vi "REQ full lifecycle.vi"(0 "ZMQ endpoint":string="tcp://127.0.0.1:5555", 1 "Julia user functions script":path=path "dummy.jl", 2 "LV Client state in":T2, 5 "data to send":string="hello", 7 "ZMQ new Timeouts in":T1={"SNDTIMEO"=-1, "RCVTIMEO"=-1}, 9 "Force command":bool, 11 "error in":errorcluster, 12 "command":T3, 13 "Jl Server state in":T2) -> (3 "LV Client state out":T2, 4 "server response":string, 6 "socket out":refnum<class "zmq_socket.lvclass">, 8 "ZMQ timeouts out":cluster{"previous":T1, "current":T1}={"previous"={"SNDTIMEO"=-1, "RCVTIMEO"=-1}, "current"={"SNDTIMEO"=-1, "RCVTIMEO"=-1}}, 10 "timeout?":bool, 14 "Jl Server state out":T2, 15 "error out":errorcluster)   [LabVIEW 2018, in "LV2Julia_core.lvlib"]
doc: "This is the central piece of the package. The VI is based on Functional Global Variable pattern to keep book on the state of the Julia server and LabView client. See the available states of the \"command\" input. For some commands, the \"Force command\" must be set."
uses:
  LV2Julia_core.lvlib
  Commands.ctl
  Server or client state.ctl
  ZMQ timeouts.ctl
  <vilib>/addons/zeromq/zmq_socket.lvclass
  <vilib>/addons/zeromq/zmq_context.lvclass
  commands LV2Jl.ctl
  expected server response.ctl
  <vilib>/addons/zeromq/socket_options.ctl
  <vilib>/Utility/error.llb/Error Cluster From Error Code.vi
  ZMQ timeouts global.vi
  <vilib>/addons/zeromq/zmq_getsocketopt_int.vi
  <vilib>/ErrorRing/Error Ring.xnode
  <vilib>/addons/zeromq/zeromq.lvlib
panel:
  out "return code":i32
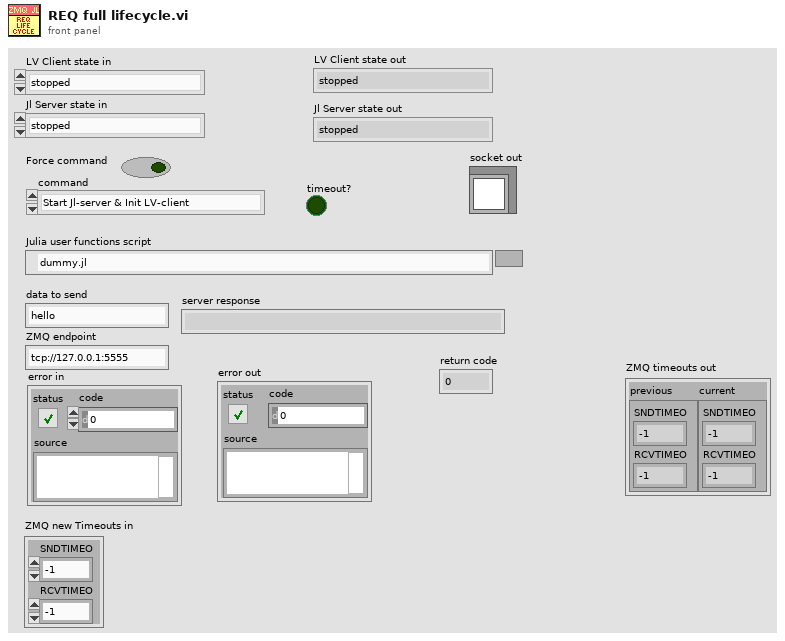
[diagram p1: front panel]
types:
  T1 = typedef "LV2Julia_core.lvlib/ZMQ timeouts.ctl" = cluster{"SNDTIMEO":i32, "RCVTIMEO":i32}
  T2 = typedef "LV2Julia_core.lvlib/Server or client state.ctl" = enum16{"stopped", "running", "unknown"}
  T3 = typedef "LV2Julia_core.lvlib/Commands.ctl" = enum16{"Start Jl-server & Init LV-client", "Send request & Get response ", "Stop Jl-server & Cleanup LV-client", "Cleanup LV-client", "Start Jl-server", "Stop Jl-server", "Init LV-Client", "Cleanup LV-Client", "(not allowed)", "Set LV Client state", "Set Jl Server state", "set ZMQ timeout", "read ZMQ timeout", "read-out state"}
  T4 = typedef "zeromq.lvlib/socket_options.ctl" = enum8{"NONE", "ZMQ_HWM", "<2>", "ZMQ_SWAP", "ZMQ_AFFINITY", "ZMQ_IDENTITY", "ZMQ_SUBSCRIBE", "ZMQ_UNSUBSCRIBE", "ZMQ_RATE", "ZMQ_RECOVERY_IVL", "ZMQ_MCAST_LOOP", "ZMQ_SNDBUF", "ZMQ_RCVBUF", "ZMQ_RCVMORE", "ZMQ_FD", "ZMQ_EVENTS", "ZMQ_TYPE", "ZMQ_LINGER", "ZMQ_RECONNECT_IVL", "ZMQ_BACKLOG", "ZMQ_RECOVERY_IVL_MSEC", "ZMQ_RECONNECT_IVL_MAX", "ZMQ_MAXMSGSIZE", "ZMQ_SNDHWM", "ZMQ_RCVHWM", "ZMQ_MULTICAST_HOPS", "<26>", "ZMQ_RCVTIMEO", "ZMQ_SNDTIMEO", "<29>", "<30>", "ZMQ_IPV4ONLY", "ZMQ_LAST_ENDPOINT", "ZMQ_ROUTER_MANDATORY", "ZMQ_TCP_KEEPALIVE", "ZMQ_TCP_KEEPALIVE_CNT", "ZMQ_TCP_KEEPALIVE_IDLE", "ZMQ_TCP_KEEPALIVE_INTVL", "ZMQ_TCP_ACCEPT_FILTER", "ZMQ_DELAY_ATTACH_ON_CONNECT", "ZMQ_XPUB_VERBOSE"}
  T5 = typedef "LV2Julia_core.lvlib/expected server response.ctl" = u16
  T6 = typedef "LV2Julia_core.lvlib/commands LV2Jl.ctl" = u8
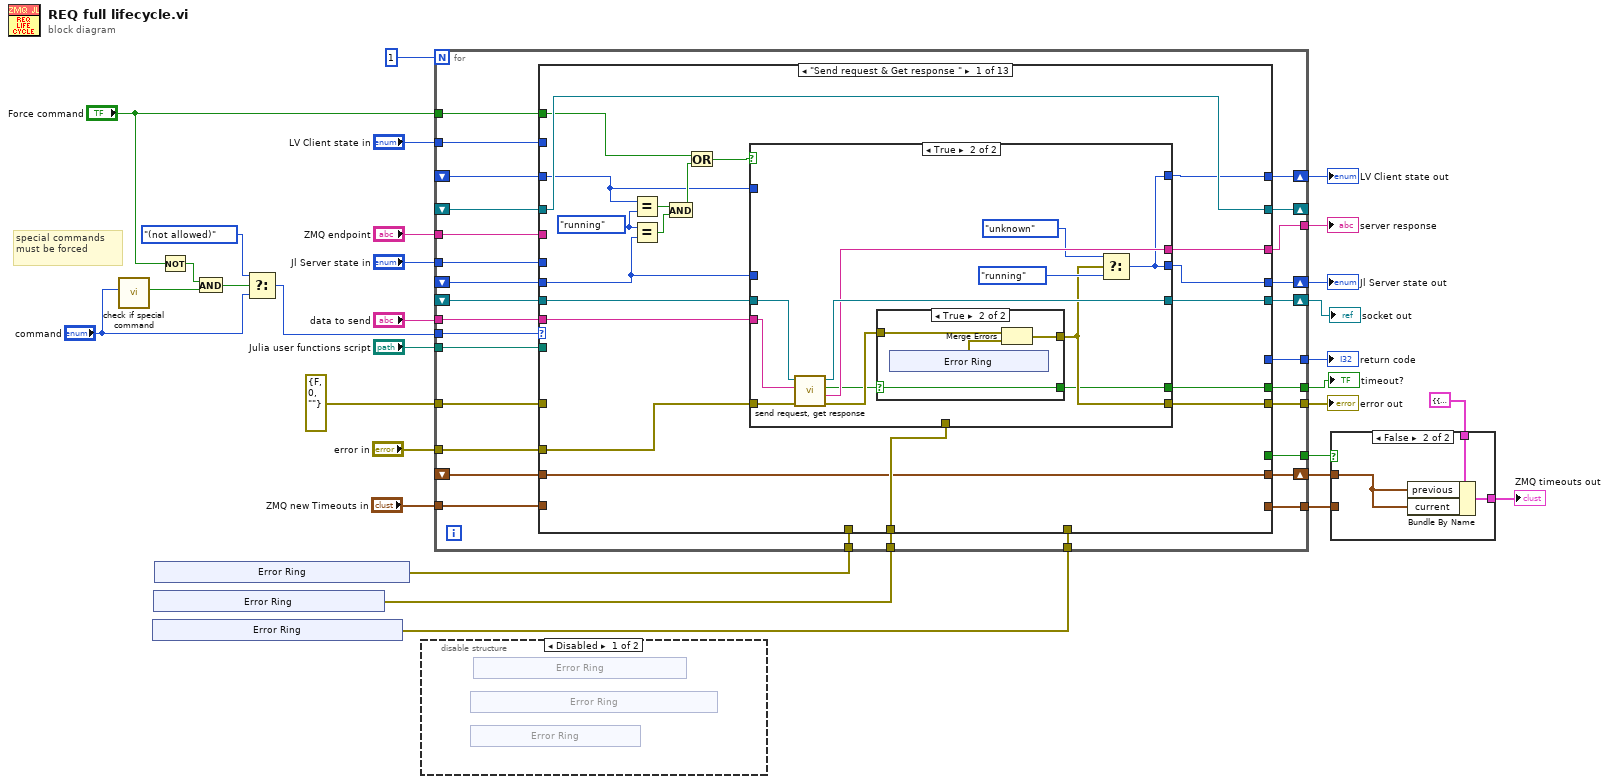
[diagram p0: block diagram]
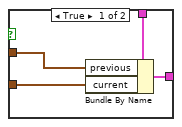
[diagram p2: hidden frame]
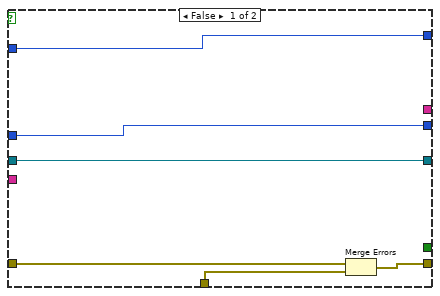
[diagram p4: hidden frame]
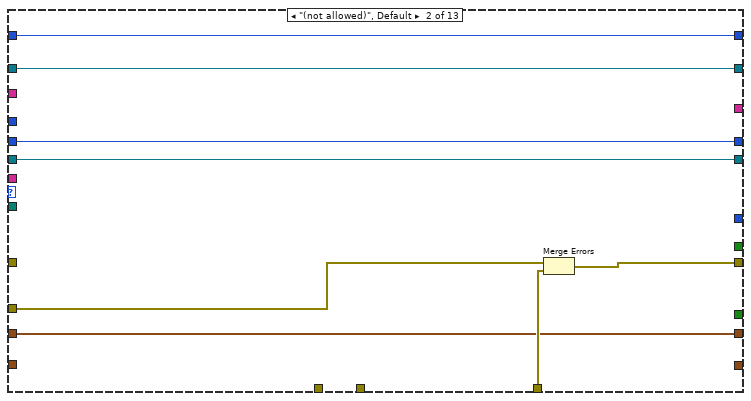
[diagram p6: hidden frame]
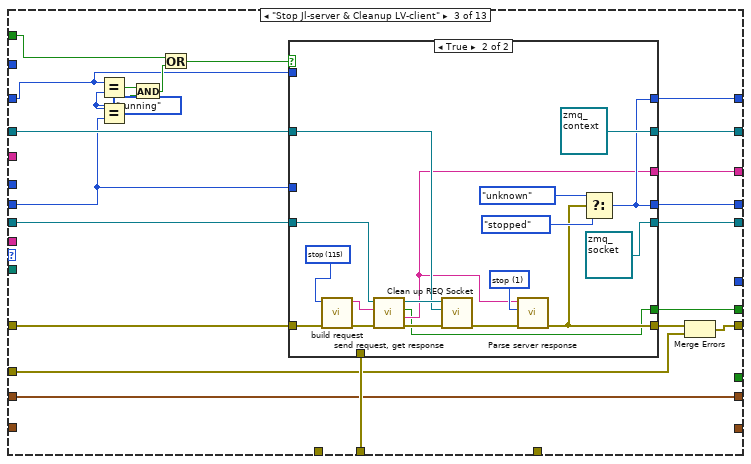
[diagram p7: hidden frame]
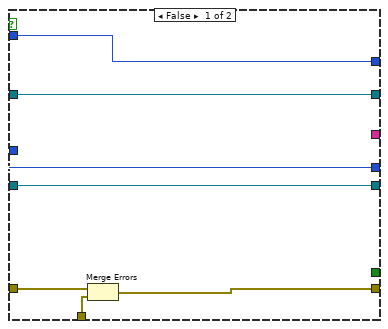
[diagram p8: hidden frame]
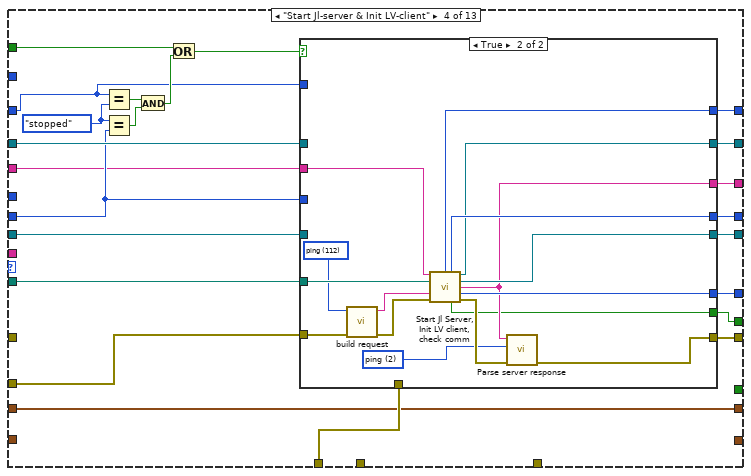
[diagram p9: hidden frame]
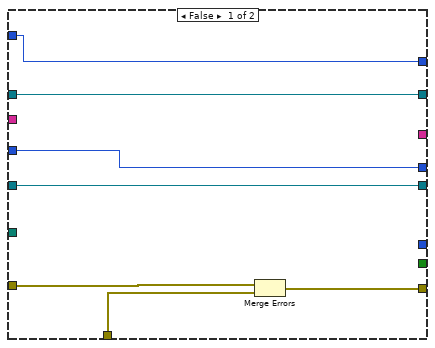
[diagram p10: hidden frame]
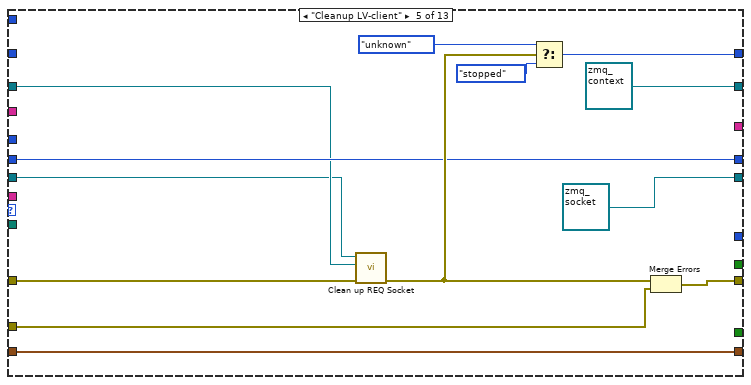
[diagram p11: hidden frame]
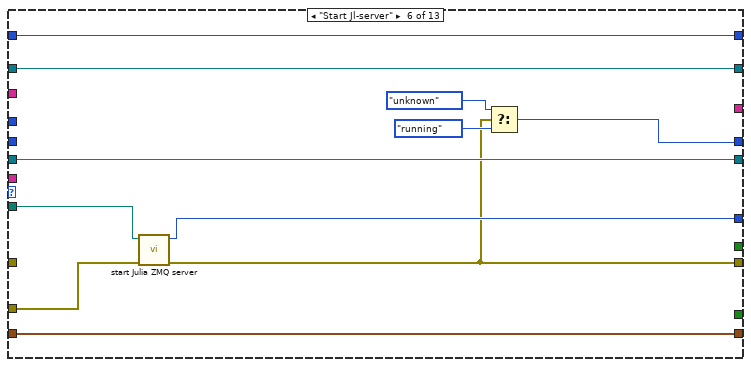
[diagram p12: hidden frame]
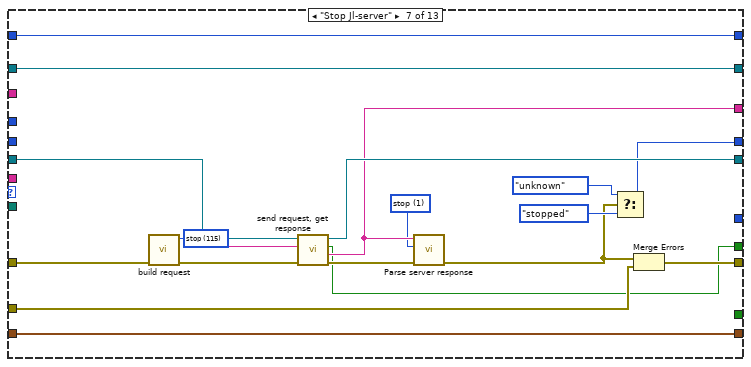
[diagram p13: hidden frame]
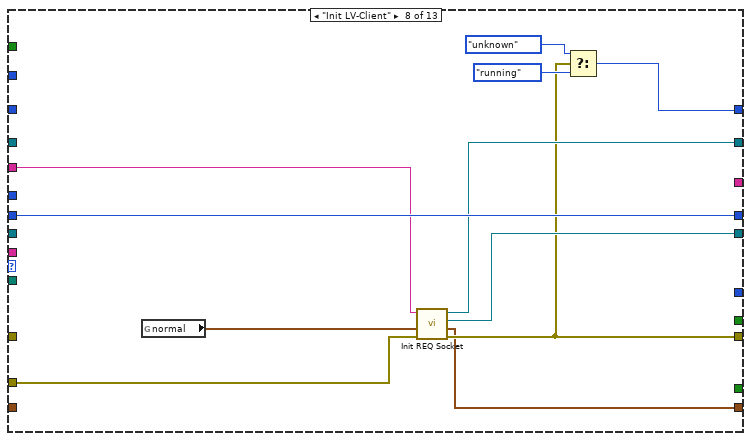
[diagram p14: hidden frame]
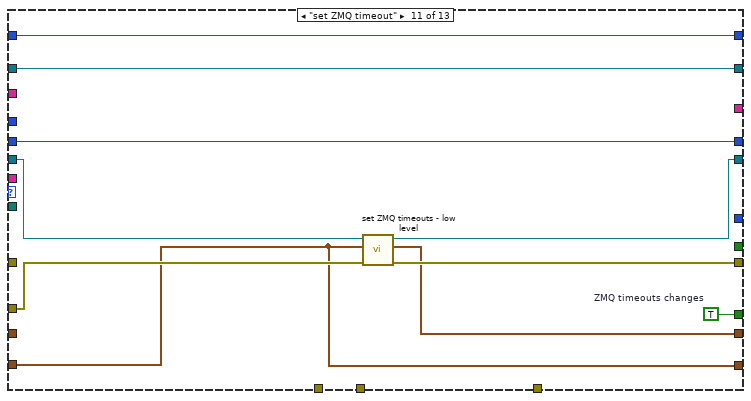
[diagram p17: hidden frame]
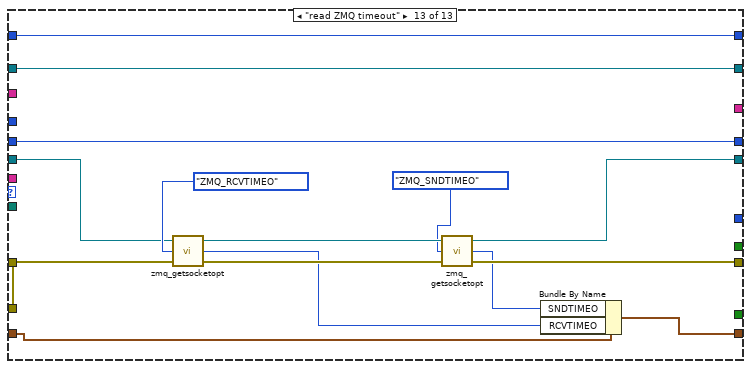
[diagram p19: hidden frame]
diagram:
  # "special commands must be forced"
  n1 = call "check if special command.vi"("command"="command") -> ("is special CMD"=w6:bool)  [unwired: 10 in]
  n2 = xnode "Error Ring"() -> ("error out"=w16:errorcluster)
  n3 = xnode "Error Ring"() -> ("error out"=w22:errorcluster)
  n4 = xnode "Error Ring"() -> ("error out"=w24:errorcluster)
  n5 = Not(x="Force command") -> (.not. x?=w20:bool)
  n6 = And(x=w20, y=w6) -> (x .and. y?=w19:bool)
  n7 = Select(t=Commands."(not allowed)" ("command"), s=w19, f="command") -> (s? t:f=w17:T3)
  n8 = disable-structure shown="Disabled" {
    frame Disabled {
      n9 = xnode "Error Ring"() -> ()  [unwired: 1 out]
      n10 = xnode "Error Ring"() -> ()  [unwired: 1 out]
      n11 = xnode "Error Ring"() -> ()  [unwired: 1 out]
    }
    frame Enabled {
    }
  }
  n12 = for {
    N: 1 -> [_]
    tunnel: [w75] -> w30
    tunnel: [w74] -> w29
    shift-right: [w73] -> _
    shift-left: _ -> [w66]
    tunnel: "ZMQ endpoint" -> [w72]
    tunnel: "data to send" -> [w71]
    shift-right: [w70] -> w9
    shift-left: _ -> [w65]
    tunnel: "error in" -> [w69]
    shift-right: [w67] -> w23
    shift-left: _ -> [w68]
    tunnel: w17 -> [w64]
    tunnel: "Julia user functions script" -> [w63]
    tunnel: w24 -> [w62]
    tunnel: "Force command" -> [w61]
    shift-right: [w60] -> w15
    shift-left: _ -> [w59]
    tunnel: w22 -> [w58]
    tunnel: w16 -> [w57]
    tunnel: [w56] -> w14
    tunnel: "LV Client state in" -> [w55]
    tunnel: "Jl Server state in" -> [w54]
    tunnel: errorcluster {"status"=FALSE, "code"=0, "source"=""} ("error in") -> [w53]
    tunnel: "ZMQ new Timeouts in" -> [w52]
    tunnel: [w50] -> w8
    shift-right: [w51] -> w4
    shift-left: _ -> [w49]
    tunnel: [w48] -> w3
    tunnel: [w47] -> w2
    n13 = case shown="\"Send request & Get response \"" w64 {
      tunnel: [w89 w131 w137 w201 w229 w241 w258 w272 w282 w288 w298 w302 w316] -> w75
      tunnel: [w90 _ w153 w190 _ _ w253 _ _ _ _ _ _] -> w74
      tunnel: [w95 w128 w148 w198 refnum<class "zmq_context.lvclass"> refnum ("zmq_context out") w246 w266 w274 w285 w290 w300 w306 w321] -> w73
      tunnel: w72 -> [_ _ _ w189 _ _ _ w271 _ _ _ _ _]
      tunnel: w71 -> [w91 _ _ _ _ _ _ _ _ _ _ _ _]
      tunnel: [w93 w126 w149 w194 refnum<class "zmq_socket.lvclass"> refnum ("zmq_socket out") w245 w265 w273 w283 w289 w295 w304 w317] -> w70
      tunnel: w69 -> [w94 w132 w136 w202 w227 w248 w256 w275 w282 w288 w297 w302 w314]
      tunnel: [w88 w127 w152 w197 w234 w242 w262 w277 w284 w287 w299 w305 w320] -> w67
      tunnel: w63 -> [_ _ _ w196 _ w239 _ _ _ _ _ _ _]
      tunnel: w65 -> [w92 w126 w154 w195 w232 w245 w268 _ w283 w289 w294 w304 w309]
      tunnel: w66 -> [w95 w128 w150 w199 w233 w246 w266 _ w285 w290 w300 w306 w321]
      tunnel: w68 -> [w79 w127 w141 w193 w234 _ _ w277 w284 _ w299 w305 w320]
      tunnel: w62 -> [_ _ _ w200 _ _ _ _ _ _ _ _ _]
      tunnel: w61 -> [w82 _ w142 w191 _ _ _ _ _ _ _ _ _]
      tunnel: [w87 w129 w140 w188 w235 w249 w267 w276 w281 w291 w301 w307 w322] -> w60
      tunnel: w59 -> [w80 w129 w138 w183 _ w249 w267 _ _ w291 w301 w307 w322]
      tunnel: w58 -> [w78 _ w139 _ _ _ _ _ _ _ _ _ _]
      tunnel: w57 -> [_ w130 _ _ _ _ _ _ _ _ _ _ _]
      tunnel: [_ _ _ w182 _ w247 _ _ _ _ _ _ _] -> w56
      tunnel: w55 -> [_ _ _ _ _ _ _ _ w281 _ _ _ _]
      tunnel: w54 -> [_ _ _ _ _ _ _ _ _ w287 _ _ _]
      tunnel: w53 -> [_ _ w135 _ w228 _ w257 _ _ _ _ _ _]
      tunnel: w52 -> [_ _ _ _ _ _ _ _ _ _ w292 _ _]
      tunnel: [w76 w125 w133 w180 w226 w240 w250 w270 w280 w286 w296 w303 w312] -> w51
      tunnel: [w77 _ w134 w181 _ _ w251 _ _ _ _ _ _] -> w50
      tunnel: w49 -> [w76 w125 w133 w180 w226 w240 w250 _ w280 w286 _ w303 w308]
      tunnel: [_ _ _ _ _ _ _ _ _ _ w293 _ _] -> w47
      tunnel: [_ _ _ _ _ _ _ _ _ _ w292 _ _] -> w48
      frame "Send request & Get response " {
        w85 = Server_or_client_state."running" ("Server state")
        n14 = Equal?(x=w80, y=w85) -> (x = y?=w83:bool)
        n15 = Equal?(x=w85, y=w79) -> (x = y?=w86:bool)
        n16 = And(x=w83, y=w86) -> (x .and. y?=w84:bool)
        n17 = Or(x=w82, y=w84) -> (x .or. y?=w81:bool)
        n18 = case shown="True" w81 {
          tunnel: w94 -> [w98 w113]
          tunnel: [w99 w112] -> w93
          tunnel: w92 -> [w99 w111]
          tunnel: w91 -> [_ w110]
          tunnel: [_ w109] -> w90
          tunnel: [w97 w104] -> w89
          tunnel: [w100 w106] -> w88
          tunnel: w79 -> [w100 _]
          tunnel: [w101 w106] -> w87
          tunnel: w80 -> [w101 _]
          tunnel: w78 -> [w96 _]
          tunnel: [_ w102] -> w77
          frame False {
            n19 = Merge Errors(w98, w96) -> (w97:errorcluster)
          }
          frame True {
            n20 = call "send request, get response.vi"("error in (no error)"=w113, "request"=w110, "zmq_socket in"=w111) -> ("error out"=w107:errorcluster, "response"=w109:string, "timeout?"=w103:bool, "zmq_socket out"=w112:refnum<class "zmq_socket.lvclass">)  [unwired: 4 in, 1 out]
            n21 = case shown="True" w103 {
              selector: w103 -> [w114 w116]
              tunnel: w107 -> [w115 w119]
              tunnel: [w115 w118] -> w104
              tunnel: [w114 w116] -> w102
              frame False {
              }
              frame True {
                n22 = xnode "Error Ring"() -> ("error out"=w117:errorcluster)
                n23 = Merge Errors(w119, w117) -> (w118:errorcluster)
              }
            }
            n24 = Select(t=Server_or_client_state."unknown" ("Server state"), s=w104, f=Server_or_client_state."running" ("Server state")) -> (s? t:f=w106:T2)
          }
        }
      }
      frame "(not allowed)", Default {
        n25 = Merge Errors(w132, w130) -> (w131:errorcluster)
      }
      frame "Stop Jl-server & Cleanup LV-client" {
        w146 = Server_or_client_state."running" ("Server state")
        n26 = Equal?(x=w138, y=w146) -> (x = y?=w144:bool)
        n27 = Equal?(x=w146, y=w141) -> (x = y?=w147:bool)
        n28 = And(x=w144, y=w147) -> (x .and. y?=w145:bool)
        n29 = Or(x=w142, y=w145) -> (x .or. y?=w143:bool)
        n30 = case shown="True" w143 {
          tunnel: w135 -> [w157 w170]
          tunnel: w154 -> [w159 w179]
          tunnel: [_ w163] -> w153
          tunnel: [w161 w172] -> w152
          tunnel: [w156 w164] -> w151
          tunnel: w150 -> [w158 w167]
          tunnel: [w159 refnum<class "zmq_socket.lvclass"> refnum ("zmq_socket out")] -> w149
          tunnel: [w158 refnum<class "zmq_context.lvclass"> refnum ("zmq_context out")] -> w148
          tunnel: w141 -> [w161 _]
          tunnel: [w160 w172] -> w140
          tunnel: w138 -> [w160 _]
          tunnel: w139 -> [w155 _]
          tunnel: [_ w162] -> w134
          frame False {
            n31 = Merge Errors(w157, w155) -> (w156:errorcluster)
          }
          frame True {
            w166 = T5 1 items=["detailed response", "stop", "ping"] ("expected response")
            w169 = T6 115 items=["call function"=99, "ping"=112, "stop"=115] ("Command")
            n32 = call "build request.vi"("error in (no error)"=w170, "Command"=w169) -> ("error out"=w171:errorcluster, "REQ string"=w168:string)  [unwired: 8 in]
            n33 = call "send request, get response.vi"("error in (no error)"=w171, "request"=w168, "zmq_socket in"=w179) -> ("error out"=w177:errorcluster, "response"=w163:string, "timeout?"=w162:bool, "zmq_socket out"=w175:refnum<class "zmq_socket.lvclass">)  [unwired: 4 in, 1 out]
            n34 = call "Clean up REQ Socket.vi"("error in (no error)"=w177, "zmq_context in"=w167, "zmq_socket in"=w175) -> ("error out"=w165:errorcluster)  [unwired: 8 in]
            n35 = call "Parse server response.vi"("error in (no error)"=w165, "expected response"=w166, "server response in"=w163) -> ("error out"=w164:errorcluster)  [unwired: 1 in, 7 out]
            n36 = Select(t=Server_or_client_state."unknown" ("Server state"), s=w164, f=Server_or_client_state."stopped") -> (s? t:f=w172:T2)
          }
        }
        n37 = Merge Errors(w151, w136) -> (w137:errorcluster)
      }
      frame "Start Jl-server & Init LV-client" {
        w186 = Server_or_client_state."stopped" ("Server state")
        n38 = Equal?(x=w183, y=w186) -> (x = y?=w184:bool)
        n39 = Equal?(x=w186, y=w193) -> (x = y?=w187:bool)
        n40 = And(x=w184, y=w187) -> (x .and. y?=w185:bool)
        n41 = Or(x=w191, y=w185) -> (x .or. y?=w192:bool)
        n42 = case shown="True" w192 {
          tunnel: w202 -> [w209 w217]
          tunnel: [w208 w213] -> w201
          tunnel: w200 -> [w207 _]
          tunnel: [w206 w222] -> w198
          tunnel: w199 -> [w206 _]
          tunnel: [w205 w223] -> w197
          tunnel: w193 -> [w205 _]
          tunnel: w196 -> [_ w225]
          tunnel: [w204 w221] -> w194
          tunnel: w195 -> [w204 _]
          tunnel: [_ w212] -> w190
          tunnel: w189 -> [_ w224]
          tunnel: [w203 w220] -> w188
          tunnel: w183 -> [w203 _]
          tunnel: [_ w219] -> w182
          tunnel: [_ w210] -> w181
          frame False {
            n43 = Merge Errors(w209, w207) -> (w208:errorcluster)
          }
          frame True {
            w211 = T5 2 items=["detailed response", "stop", "ping"] ("expected response")
            w216 = T6 112 items=["call function"=99, "ping"=112, "stop"=115] ("Command")
            n44 = call "build request.vi"("error in (no error)"=w217, "Command"=w216) -> ("error out"=w218:errorcluster, "REQ string"=w215:string)  [unwired: 8 in]
            n45 = call "Start Jl Server, Init LV client, check comm.vi"("endpoint"=w224, "Julia user functions script"=w225, "request"=w215, "error in (no error)"=w218) -> ("LV client state"=w220:T2, "JL server state"=w223:T2, "zmq_context out"=w222:refnum<class "zmq_context.lvclass">, "zmq_socket out"=w221:refnum<class "zmq_socket.lvclass">, "response"=w212:string, "script return code (0)"=w219:i32, "timeout?"=w210:bool, "error out"=w214:errorcluster)  [unwired: 2 in, 2 out]
            n46 = call "Parse server response.vi"("error in (no error)"=w214, "expected response"=w211, "server response in"=w212) -> ("error out"=w213:errorcluster)  [unwired: 1 in, 7 out]
          }
        }
      }
      frame "Cleanup LV-client" {
        n47 = call "Clean up REQ Socket.vi"("error in (no error)"=w228, "zmq_context in"=w233, "zmq_socket in"=w232) -> ("error out"=w236:errorcluster)  [unwired: 8 in]
        n48 = Select(t=Server_or_client_state."unknown" ("Server state"), s=w236, f=Server_or_client_state."stopped") -> (s? t:f=w235:T2)
        n49 = Merge Errors(w236, w227) -> (w229:errorcluster)
      }
      frame "Start Jl-server" {
        n50 = call "start Julia ZMQ server.vi"("error in (no error)"=w248, "Julia user functions script"=w239) -> ("error out"=w241:errorcluster, "return code"=w247:i32)  [unwired: 6 in, 2 out]
        n51 = Select(t=Server_or_client_state."unknown" ("Server state"), s=w241, f=Server_or_client_state."running") -> (s? t:f=w242:T2)
      }
      frame "Stop Jl-server" {
        w252 = T5 1 items=["detailed response", "stop", "ping"] ("expected response")
        w260 = T6 115 items=["call function"=99, "ping"=112, "stop"=115] ("Command")
        n52 = call "build request.vi"("error in (no error)"=w257, "Command"=w260) -> ("error out"=w261:errorcluster, "REQ string"=w259:string)  [unwired: 8 in]
        n53 = call "send request, get response.vi"("error in (no error)"=w261, "request"=w259, "zmq_socket in"=w268) -> ("error out"=w255:errorcluster, "response"=w253:string, "timeout?"=w251:bool, "zmq_socket out"=w265:refnum<class "zmq_socket.lvclass">)  [unwired: 4 in, 1 out]
        n54 = call "Parse server response.vi"("error in (no error)"=w255, "expected response"=w252, "server response in"=w253) -> ("error out"=w254:errorcluster)  [unwired: 1 in, 7 out]
        n55 = Select(t=Server_or_client_state."unknown" ("Server state"), s=w254, f=Server_or_client_state."stopped") -> (s? t:f=w262:T2)
        n56 = Merge Errors(w254, w256) -> (w258:errorcluster)
      }
      frame "Init LV-Client" {
        n57 = global read "ZMQ timeouts global.vi" "normal"() -> (w269:T1)
        n58 = call "Init REQ Socket.vi"("error in (no error)"=w275, "ZMQ new Timeouts in"=w269, "endpoint"=w271) -> ("error out"=w272:errorcluster, "ZMQ new Timeouts out"=w270:T1, "socket out"=w273:refnum<class "zmq_socket.lvclass">, "zmq_context out"=w274:refnum<class "zmq_context.lvclass">)  [unwired: 5 in]
        n59 = Select(t=Server_or_client_state."unknown" ("Server state"), s=w272, f=Server_or_client_state."running") -> (s? t:f=w276:T2)
      }
      frame "Set LV Client state" {
      }
      frame "Set Jl Server state" {
      }
      frame "set ZMQ timeout" {
        w293 = TRUE  # ZMQ timeouts changes
        n60 = call "set ZMQ timeouts - low level.vi"("error in (no error)"=w297, "ZMQ new Timeouts in"=w292, "zmq_socket in"=w294) -> ("error out"=w298:errorcluster, "ZMQ new Timeouts out"=w296:T1, "zmq_socket out"=w295:refnum<class "zmq_socket.lvclass">)  [unwired: 6 in]
      }
      frame "read-out state" {
      }
      frame "read ZMQ timeout" {
        n61 = call-poly <vilib>:"zmq_getsocketopt.vi"("error in"=w314, "option"=socket_options."ZMQ_RCVTIMEO", "socket in"=w309) -> ("error out"=w319:errorcluster, "value"=w311:i32, "socket out"=w318:refnum<class "zmq_socket.lvclass">)
        n62 = call-poly <vilib>:"zmq_getsocketopt.vi"("error in"=w319, "option"=socket_options."ZMQ_SNDTIMEO", "socket in"=w318) -> ("error out"=w316:errorcluster, "value"=w310:i32, "socket out"=w317:refnum<class "zmq_socket.lvclass">)
        n63 = Bundle By Name(cluster=w308, "SNDTIMEO"=w310, "RCVTIMEO"=w311) -> (w312:T1)
      }
    }
  }
  "error out" <- w30
  "server response" <- w29
  "Jl Server state out" <- w23
  "LV Client state out" <- w15
  "return code" <- w14
  "socket out" <- w9
  "timeout?" <- w8
  n64 = case shown="False" w2 {
    tunnel: [w326 w329] -> w5
    tunnel: w4 -> [w325 w327]
    tunnel: w3 -> [w324 _]
    tunnel: cluster{"previous":T1, "current":T1} {"previous"={"SNDTIMEO"=-1, "RCVTIMEO"=-1}, "current"={"SNDTIMEO"=-1, "RCVTIMEO"=-1}} ("ZMQ timeouts out") -> [w323 w328]
    frame True {
      n65 = Bundle By Name(cluster=w323, "previous"=w325, "current"=w324) -> (w326:cluster{"previous":T1, "current":T1})
    }
    frame False {
      n66 = Bundle By Name(cluster=w328, "previous"=w327, "current"=w327) -> (w329:cluster{"previous":T1, "current":T1})
    }
  }
  "ZMQ timeouts out" <- w5
